vi "Write Path Cluster.vi"(8 "error in (no error)":errorcluster, 10 "Path Cluster":cluster{"Numeric":dbl}, 11 "Setting Database in":refnum<class "Setting Database.lvclass">) -> (0 "error out":errorcluster, 3 "Setting Database out":refnum<class "Setting Database.lvclass">)   [LabVIEW 2020]
uses:
  Setting Database.lvclass
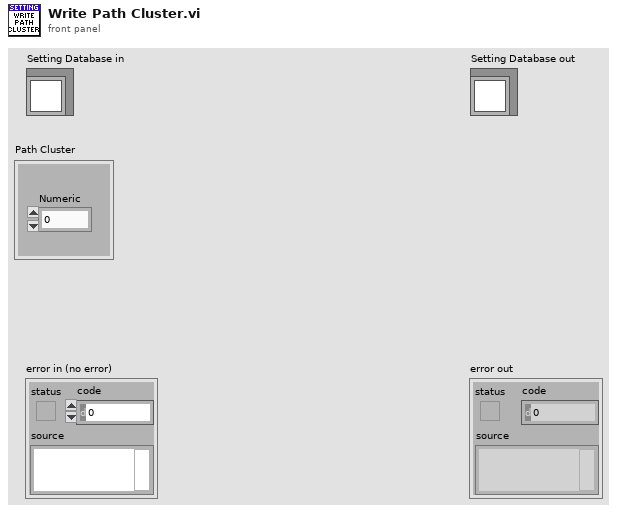
[diagram p1: front panel]
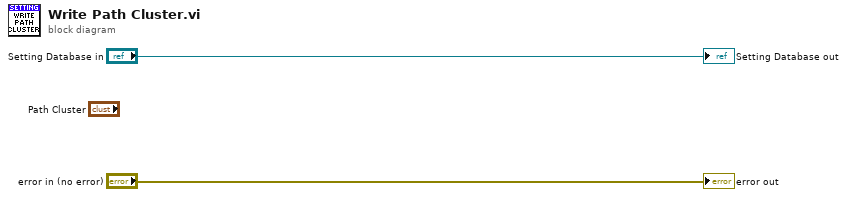
[diagram p0: block diagram]
diagram:
  "error out" <- "error in (no error)"
  "Setting Database out" <- "Setting Database in"
